vi "NaN operations.vi"(3 "Data(in)":dbl[](array[numeric]) format="%.2f", 5 "Operation":enum16{"Remove NaNs", "Convert -inf to NaN"}(ring)) -> (0 "Data(out)":dbl[](array[numeric]) format="%.2f")   [LabVIEW 2013, in "nan operations.lvlib"]
uses:
  nan operations.lvlib
panel:
  # "Copyright Americo A. Migliaccio (c) 2002 All Rights Reserved by Author"
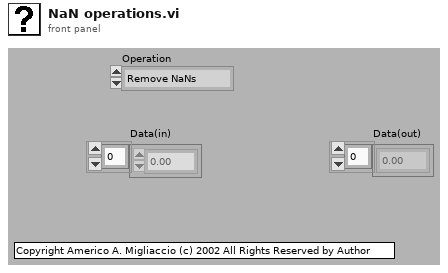
[diagram p1: front panel]
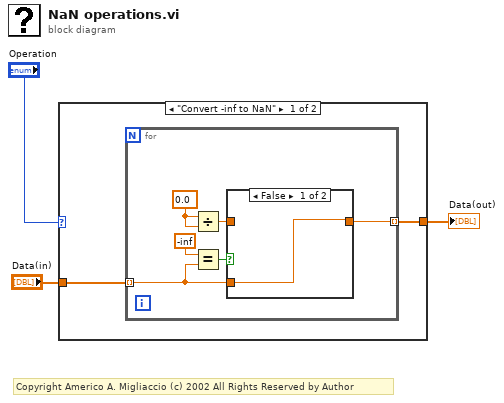
[diagram p0: block diagram]
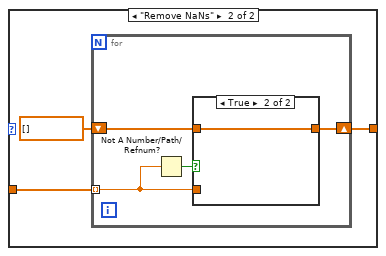
[diagram p3: hidden frame]
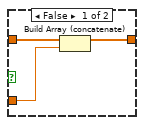
[diagram p4: hidden frame]
diagram:
  # "Copyright Americo A. Migliaccio (c) 2002 All Rights Reserved by Author"
  n1 = case shown="\"Convert -inf to NaN\"" "Operation" {
    tunnel: "Data(in)" -> [w5 w16]
    tunnel: [w4 w15] -> w1
    frame "Convert -inf to NaN" {
      n2 = for {
        tunnel: w5 -> [w7] mode=indexing
        tunnel: [w6] -> w4 mode=indexing
        w9 = 0.0 ("x")
        n3 = Divide(x=w9, y=w9) -> (x/y=w8:dbl)
        n4 = Equal?(x=-inf, y=w7) -> (x = y?=w10:bool)
        n5 = case shown="False" w10 {
          tunnel: w8 -> [_ w13]
          tunnel: [w12 w13] -> w6
          tunnel: w7 -> [w12 _]
          frame False {
          }
          frame True {
          }
        }
      }
    }
    frame "Remove NaNs" {
      n6 = for {
        tunnel: w16 -> [w17] mode=indexing
        shift-right: [w19] -> w15
        shift-left: dbl[] [] -> [w18]
        n7 = Not A Number/Path/Refnum?(number/path/refnum=w17) -> (NaN/Path/Refnum?=w20:bool)
        n8 = case shown="True" w20 {
          tunnel: [w23 w24] -> w19
          tunnel: w18 -> [w22 w24]
          tunnel: w17 -> [w21 _]
          frame False {
            n9 = Build Array (concatenate)(w22, w21) -> (w23:dbl[])
          }
          frame True {
          }
        }
      }
    }
  }
  "Data(out)" <- w1
